vi "NI VeriStand - Lock Connection.vi"(8 "error in (no error)":errorcluster, 9 "New Password":string, 10 "Old Password (\"\")":string, 11 "WorkspaceManager in":T1) -> (0 "error out":errorcluster, 3 "WorkspaceManager out":T1)   [LabVIEW 2020, in "NI_VS Workspace ExecutionAPI.lvlib"]
doc: "Locks the current VeriStand Gateway connection. If the connection already is locked, you must provide the current password in order to set a new one."
uses:
  <vilib>/NI VeriStand/Execution/Workspace/NI_VS Workspace ExecutionAPI.lvlib
  <vilib>/NI VeriStand/Execution/Workspace/WorkspaceAPI.ctl
  NationalInstruments.VeriStand.ClientAPI
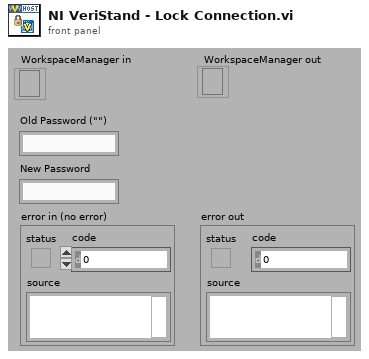
[diagram p1: front panel]
types:
  T1 = typedef "NI_VS Workspace ExecutionAPI.lvlib/WorkspaceAPI.ctl" = refnum<k24>
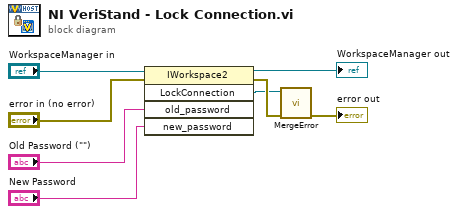
[diagram p0: block diagram]
diagram:
  n1 = invoke class="IWorkspace2" method="LockConnection"(reference="WorkspaceManager in", error in="error in (no error)", "old_password"="Old Password (\"\")", "new_password"="New Password") -> (reference out=→"WorkspaceManager out":T1, error out=w8:errorcluster, "LockConnection"=w3:refnum<k24>)  [unwired: 1 in, 2 out]
  n2 = call <vilib>:"MergeError.vi"("error in (no error)"=w8, "Error"=w3) -> ("error out"=→"error out":errorcluster)  [unwired: 9 out]
